vi "Split JSON String.vi"(8 "error in (no error)":errorcluster, 11 "string":string) -> (0 "error out":errorcluster, 1 "dsf configuration substring":string, 2 "dsf version substring":string, 3 "file version substring":string)   [LabVIEW 2017, in "DSF Core.lvlib" / "Configuration Session.lvclass"]
uses:
  Configuration Session.lvclass
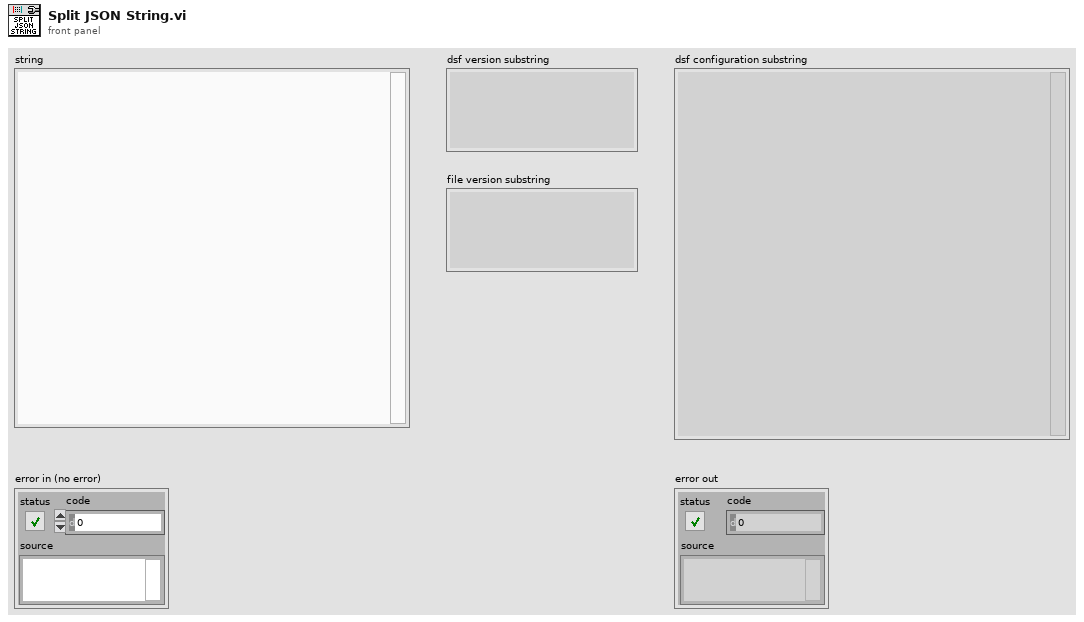
[diagram p1: front panel]
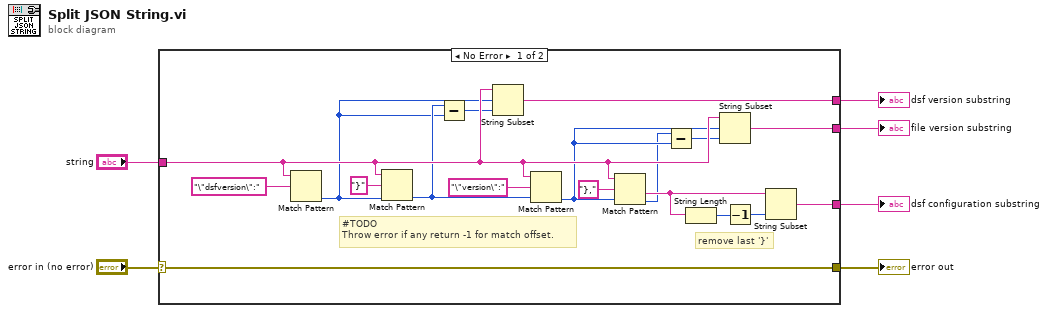
[diagram p0: block diagram]
diagram:
  n1 = case shown="No Error" "error in (no error)" {
    selector: "error in (no error)" -> [w7 w25]
    tunnel: [w18 _] -> w6
    tunnel: "string" -> [w17 _]
    tunnel: [w10 _] -> w4
    tunnel: [w9 _] -> w3
    tunnel: [w7 w25] -> w1
    frame No Error {
      # "#TODO\nThrow error if any return -1 for match offset."
      # "remove last '}'"
      n2 = Match Pattern(string=w17, regular expression="\"dsfversion\":") -> (offset past match=w12:i32)  [unwired: 1 in, 3 out]
      n3 = Match Pattern(string=w17, regular expression="}", offset (0)=w12) -> (offset past match=w13:i32)  [unwired: 3 out]
      n4 = Subtract(x=w13, y=w12) -> (x-y=w11:i32)
      n5 = String Subset(string=w17, offset (0)=w12, length (rest)=w11) -> (substring=w10:string)
      n6 = Match Pattern(string=w17, regular expression="\"version\":", offset (0)=w13) -> (offset past match=w15:i32)  [unwired: 3 out]
      n7 = Match Pattern(string=w17, regular expression="},", offset (0)=w15) -> (after substring=w20:string, offset past match=w14:i32)  [unwired: 2 out]
      n8 = Subtract(x=w14, y=w15) -> (x-y=w16:i32)
      n9 = String Length(string=w20) -> (length=w21:i32)
      n10 = String Subset(string=w17, offset (0)=w15, length (rest)=w16) -> (substring=w9:string)
      n11 = Decrement(x=w21) -> (x-1=w19:i32)
      n12 = String Subset(string=w20, length (rest)=w19) -> (substring=w18:string)  [unwired: 1 in]
    }
    frame Error {
    }
  }
  "dsf version substring" <- w4
  "dsf configuration substring" <- w6
  "file version substring" <- w3
  "error out" <- w1
